vi "ChangeToYellowLight.vi"(0 "object in":refnum<class "TrafficLight.lvclass">, 5 "Error In":errorcluster) -> (14 "object out":refnum<class "TrafficLight.lvclass">, 19 "Error Out":errorcluster)   [LabVIEW 2024, in "TrafficLight.lvclass"]
uses:
  <resource>/Framework/Providers/Open_GDS/ClassProviders/Provider_LvNativeClass/Templates/NativeBaseTemplate/NativeBaseTemplate.lvclass/NativeBaseTemplate.ctl
  TrafficLight.lvclass
  TrafficLight.lvclass/TrafficLight.ctl
panel:
  # "Connector Pane"
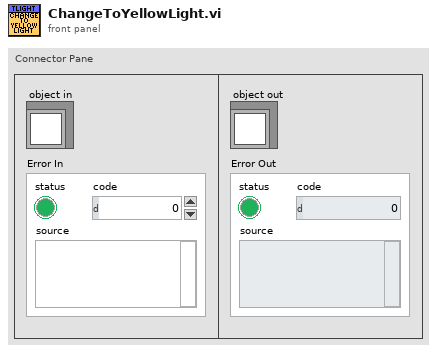
[diagram p1: front panel]
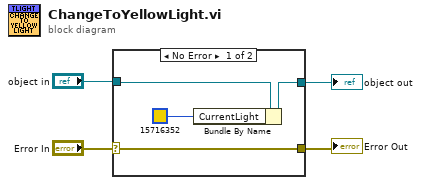
[diagram p0: block diagram]
diagram:
  n1 = case shown="No Error" "Error In" {
    selector: "Error In" -> [w8 w10]
    tunnel: [w8 w10] -> w3
    tunnel: [w6 w9] -> w1
    tunnel: "object in" -> [w7 w9]
    frame No Error {
      n2 = Bundle By Name(cluster=w7, "CurrentLight"=u32 15716352) -> (w6:refnum<class "TrafficLight.lvclass">)
    }
    frame Error {
    }
  }
  "Error Out" <- w3
  "object out" <- w1
